vi "parse_create_collection_response.vi"(0 "headers":string, 5 "body":string, 11 "error in (no error)":errorcluster) -> (15 "error out":errorcluster)   [LabVIEW 2020, in "vector_weviate.lvclass"]
uses:
  vector_weviate.lvclass
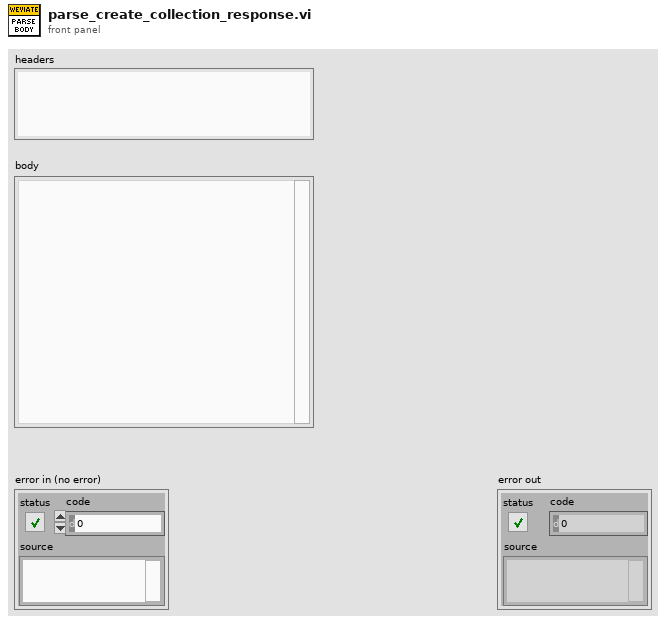
[diagram p1: front panel]
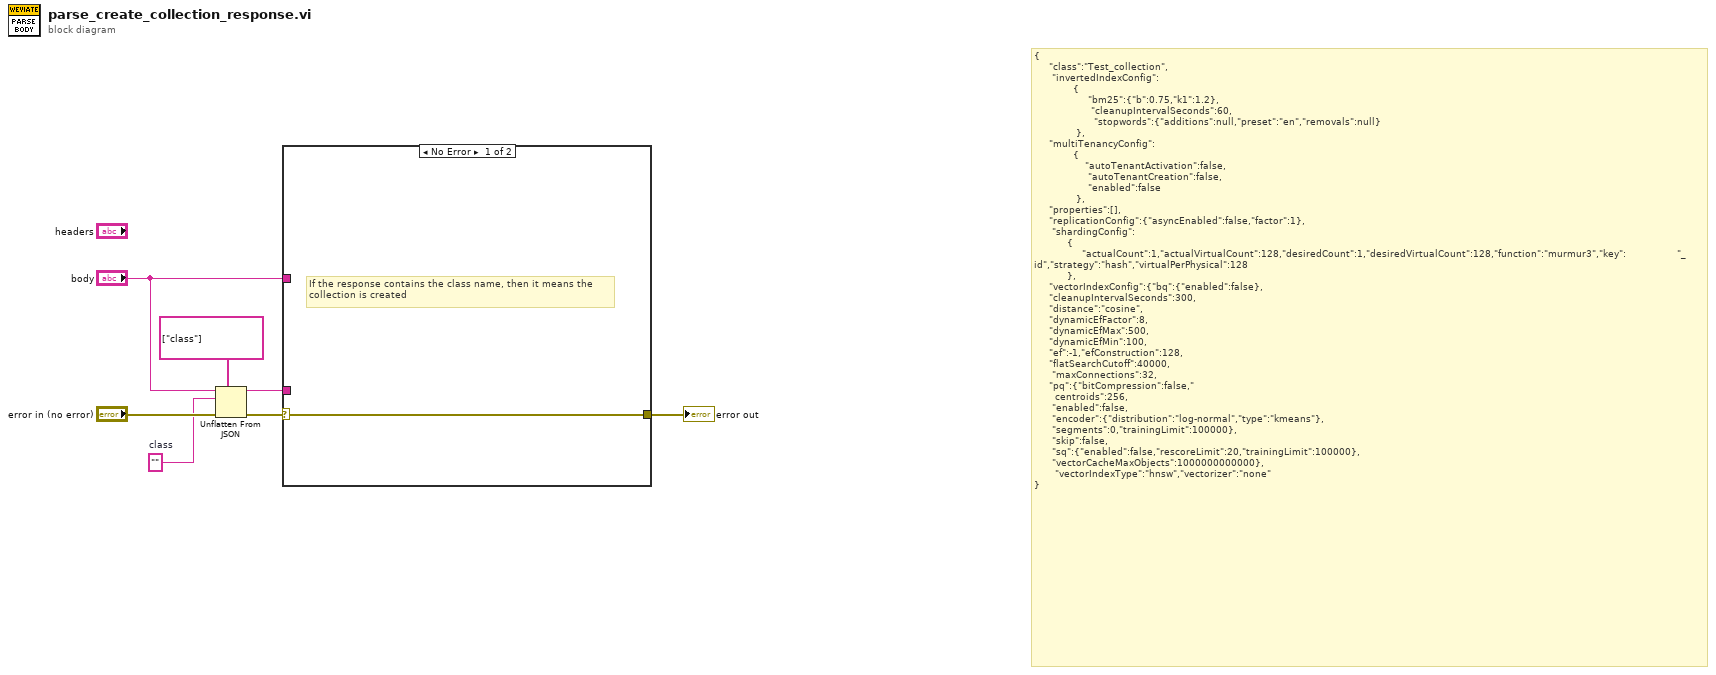
[diagram p0: block diagram]
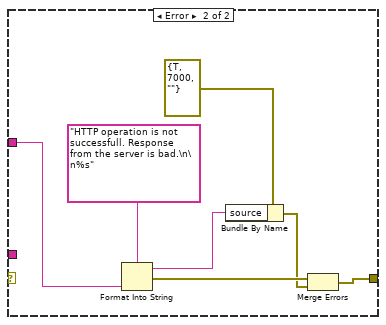
[diagram p2: hidden frame]
diagram:
  w1 = ""  # class
  # "{\n     \"class\":\"Test_collection\",\n      \"invertedIndexConfig\":\n             {\n                  \"bm25\":{\"b\":0.75,\"k1\":1.2},\n                   \"cleanupIntervalSeconds\":60,\n                    \"stopwords\":{\"additions\":null,\"preset\":\"en\",\"removals\":null}\n              },\n     \"multiTenancyConfig\":\n             {\n                 \"autoTenantActivation\":false,\n                  \"autoTenantCreation\":false,\n                  \"enabled\":false\n              },\n     \"properties\":[],\n     \"replicationConfig\":{\"asyncEnabled\":false,\"factor\":1},\n      \"shardingConfig\":\n           {\n                \"actualCount\":1,\"actualVirtualCount\":128,\"desiredCount\":1,\"desiredVirtualCount\":128,\"function\":\"murmur3\",\"key\":                 \"_id\",\"strategy\":\"hash\",\"virtualPerPhysical\":128\n           },\n     \"vectorIndexConfig\":{\"bq\":{\"enabled\":false},\n     \"cleanupIntervalSeconds\":300,\n     \"distance\":\"cosine\",\n     \"dynamicEfFactor\":8,\n     \"dynamicEfMax\":500,\n     \"dynamicEfMin\":100,\n     \"ef\":-1,\"efConstruction\":128,\n     \"flatSearchCutoff\":40000,\n      \"maxConnections\":32,\n     \"pq\":{\"bitCompression\":false,\"\n       centroids\":256,\n      \"enabled\":false,\n      \"encoder\":{\"distribution\":\"log-normal\",\"type\":\"kmeans\"},\n      \"segments\":0,\"trainingLimit\":100000},\n      \"skip\":false,\n      \"sq\":{\"enabled\":false,\"rescoreLimit\":20,\"trainingLimit\":100000},\n      \"vectorCacheMaxObjects\":1000000000000},\n       \"vectorIndexType\":\"hnsw\",\"vectorizer\":\"none\"\n}"
  n1 = Unflatten From JSON(path=string[] ["class"], JSON string="body", type and defaults=w1, error in (no error)="error in (no error)") -> (value=w4:string, error out=w5:errorcluster)  [unwired: 3 in]
  n2 = case shown="No Error" w5 {
    selector: w5 -> [w8 _]
    tunnel: w4 -> [_ _]
    tunnel: [w8 w9] -> w3
    tunnel: "body" -> [_ w12]
    frame No Error {
      # "If the response contains the class name, then it means the\ncollection is created"
    }
    frame Error {
      n3 = Format Into String(format string="HTTP operation is not successfull. Response from the server is bad.\n\n%s", w12) -> (resulting string=w14:string, error out=w11:errorcluster)  [unwired: 2 in]
      n4 = Bundle By Name(cluster=errorcluster {"status"=TRUE, "code"=7000, "source"=""} ("error constant"), "source"=w14) -> (w10:errorcluster)
      n5 = Merge Errors(w11, w10) -> (w9:errorcluster)
    }
  }
  "error out" <- w3
